vi "CFSensor2.5Kpa-SerialPortDataParse.vi"(10 "error in":errorcluster, 11 "InputStr":string) -> (2 "error out":errorcluster, 3 "OutputStr":string)   [LabVIEW 2023]
panel:
  out "PressNum":dbl=10.5556
  out "TempNum":dbl=10.5556
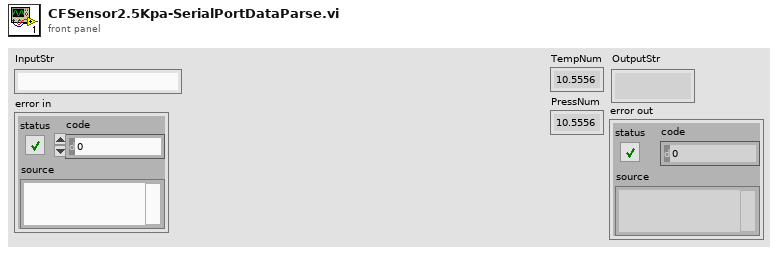
[diagram p1: front panel]
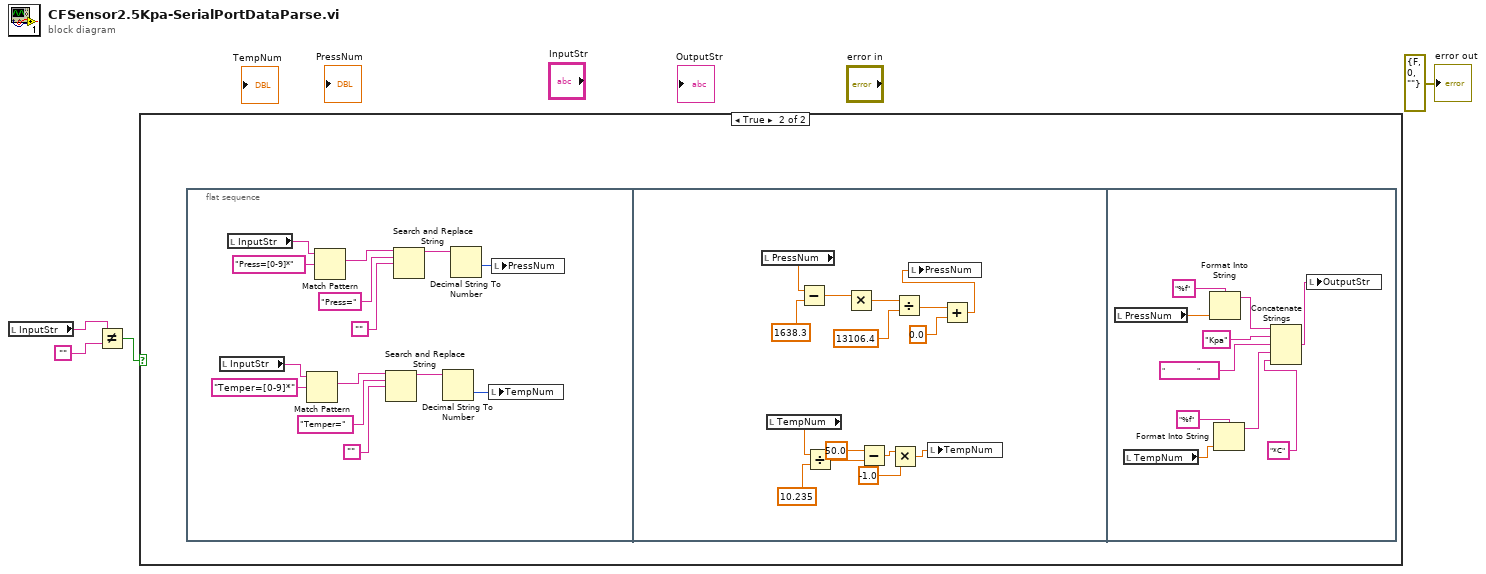
[diagram p0: block diagram]
diagram:
  n1 = local read "InputStr"() -> (w3:string)
  n2 = Not Equal?(x=w3, y="") -> (x != y?=w1:bool)
  n3 = case shown="True" w1 {
    frame False {
    }
    frame True {
      n4 = flat-sequence {
        frame #0 {
          n5 = local read "InputStr"() -> (w15:string)
          n6 = local read "InputStr"() -> (w6:string)
          n7 = Match Pattern(string=w15, regular expression="Temper=[0-9]*") -> (match substring=w14:string)  [unwired: 1 in, 3 out]
          n8 = Match Pattern(string=w6, regular expression="Press=[0-9]*") -> (match substring=w7:string)  [unwired: 1 in, 3 out]
          n9 = Search and Replace String(input string=w14, search string="Temper=", replace string="") -> (result string=w11:string)  [unwired: 5 in, 3 out]
          n10 = Search and Replace String(input string=w7, search string="Press=", replace string="") -> (result string=w10:string)  [unwired: 5 in, 3 out]
          n11 = Decimal String To Number(string=w11) -> (number=w18:i32)  [unwired: 2 in, 1 out]
          n12 = Decimal String To Number(string=w10) -> (number=w17:i32)  [unwired: 2 in, 1 out]
          n13 = local write "TempNum"(w18) -> ()
          n14 = local write "PressNum"(w17) -> ()
        }
        frame #1 {
          n15 = local read "PressNum"() -> (w25:dbl)
          n16 = local read "TempNum"() -> (w27:dbl)
          n17 = Subtract(x=w25, y=1638.3) -> (x-y=w24:dbl)
          n18 = Divide(x=w27, y=10.235) -> (x/y=w29:dbl)
          n19 = Multiply(x=w24) -> (x*y=w23:dbl)  [unwired: 1 in]
          n20 = Subtract(x=50.0, y=w29) -> (x-y=w32:dbl)
          n21 = Multiply(x=w32, y=-1.0) -> (x*y=w31:dbl)
          n22 = Divide(x=w23, y=13106.4) -> (x/y=w21:dbl)
          n23 = local write "TempNum"(w31) -> ()
          n24 = Add(x=w21, y=0.0) -> (x+y=w19:dbl)
          n25 = local write "PressNum"(w19) -> ()
        }
        frame #2 {
          n26 = local read "PressNum"() -> (w41:dbl)
          n27 = local read "TempNum"() -> (w37:dbl)
          n28 = Format Into String(format string="%f", w41) -> (resulting string=w40:string)  [unwired: 2 in, 1 out]
          n29 = Format Into String(format string="%f", w37) -> (resulting string=w36:string)  [unwired: 2 in, 1 out]
          n30 = Concatenate Strings(w40, "Kpa" ("string"), "                " ("string"), w36, "*C" ("string")) -> (w43:string)
          n31 = local write "OutputStr"(w43) -> ()
        }
      }
    }
  }
  "error out" <- errorcluster {"status"=FALSE, "code"=0, "source"=""} ("error out")
